vi "SPAN Stufen abfragen Gasteiler alle Komponenten.vi"(5 "GD LNI Cluster":T2, 6 "Sprachliste":string[][](array[string]), 7 "Boolsche Flags Cluster":T13, 8 "error in (no error)":errorcluster caption="Fehler (Eingang, kein Fehler)", 9 "Referenzen Cluster":T12, 10 "SPAN Index in":i32, 11 "SpanInletClusterArray in":T3[](array[typedef]) {"zusätzliche Zeitdauer Erster Punkt" min=30 step=1 format="%#_5g"; "Zeitdauer Stufen" format="%#_5g"; "Max Fehler" format="%#_5g"; "Anzahl Stufen" format="%#_5g"; "Komponenten"."Komponente 5"."Komponente:" items=["NO (350,3000) LP 191C", "NO2 (150) LP 191C (1of2)", "NO2 (2000) LP 191C (2of2)", "N2O (300) LP 191C (1of2)", "NH3 (300) LP 191C (1of2)", "NH3 (900,3000) LP 191C (2of2)", "HNCO (400) 191C", "H2O% (30) LP 191C", "Formaldehyde (70,500) LP 191C", "CO2 low% (4) LP 191C (2of2)", "CO2% (20) LP 191C (1of2)", "CO (700) LP 191C (1of3)", "CO% (1) LP 191C (2of3)", "Propylene (1000) LP 191C", "Aromatic HC C7 (500) LP 191C", "Ethylene (1000) LP 191C", "CH4 (250) LP 191C (1of2)", "CH4 (5000) LP 191C (2of2)", "Ethane (1000) LP 191C", "Acetylene (1000) LP 191C", "HNO2 (20) 191C", "MeOH (1000) 191C", "CO% (10) LP 191C (3of3)", "Formic Acid (100) 191C", "SO2 (500) LP 191C", "Acetaldehyde (1000) LP 191C", "COS (100) LP 191C", "1,3 butadiene (100) LP 191C", "Oil as Octane (200) LP 191C", "N2O (1000) LP 191C (2of2)", "Propane (200) LP 191C", "NO2 autorange (2000)", "CO autorange (100000)", "CH4 autorange (5000)", "NH3 autorange (3000)", "Temp. Gascell", "Pressure Gascell", "sBeam@2500"]; "Komponenten"."Komponente 5"."Konzentration IST" format="%#.4f"; "Komponenten"."Komponente 5"."Genauigkeit" format="%#.1f"; "Komponenten"."Komponente 4"."Komponente:" items=["NO (350,3000) LP 191C", "NO2 (150) LP 191C (1of2)", "NO2 (2000) LP 191C (2of2)", "N2O (300) LP 191C (1of2)", "NH3 (300) LP 191C (1of2)", "NH3 (900,3000) LP 191C (2of2)", "HNCO (400) 191C", "H2O% (30) LP 191C", "Formaldehyde (70,500) LP 191C", "CO2 low% (4) LP 191C (2of2)", "CO2% (20) LP 191C (1of2)", "CO (700) LP 191C (1of3)", "CO% (1) LP 191C (2of3)", "Propylene (1000) LP 191C", "Aromatic HC C7 (500) LP 191C", "Ethylene (1000) LP 191C", "CH4 (250) LP 191C (1of2)", "CH4 (5000) LP 191C (2of2)", "Ethane (1000) LP 191C", "Acetylene (1000) LP 191C", "HNO2 (20) 191C", "MeOH (1000) 191C", "CO% (10) LP 191C (3of3)", "Formic Acid (100) 191C", "SO2 (500) LP 191C", "Acetaldehyde (1000) LP 191C", "COS (100) LP 191C", "1,3 butadiene (100) LP 191C", "Oil as Octane (200) LP 191C", "N2O (1000) LP 191C (2of2)", "Propane (200) LP 191C", "NO2 autorange (2000)", "CO autorange (100000)", "CH4 autorange (5000)", "NH3 autorange (3000)", "Temp. Gascell", "Pressure Gascell", "sBeam@2500"]; "Komponenten"."Komponente 4"."Konzentration IST" format="%#.4f"; "Komponenten"."Komponente 4"."Genauigkeit" format="%#.1f"; "Komponenten"."Komponente 3"."Komponente:" items=["NO (350,3000) LP 191C", "NO2 (150) LP 191C (1of2)", "NO2 (2000) LP 191C (2of2)", "N2O (300) LP 191C (1of2)", "NH3 (300) LP 191C (1of2)", "NH3 (900,3000) LP 191C (2of2)", "HNCO (400) 191C", "H2O% (30) LP 191C", "Formaldehyde (70,500) LP 191C", "CO2 low% (4) LP 191C (2of2)", "CO2% (20) LP 191C (1of2)", "CO (700) LP 191C (1of3)", "CO% (1) LP 191C (2of3)", "Propylene (1000) LP 191C", "Aromatic HC C7 (500) LP 191C", "Ethylene (1000) LP 191C", "CH4 (250) LP 191C (1of2)", "CH4 (5000) LP 191C (2of2)", "Ethane (1000) LP 191C", "Acetylene (1000) LP 191C", "HNO2 (20) 191C", "MeOH (1000) 191C", "CO% (10) LP 191C (3of3)", "Formic Acid (100) 191C", "SO2 (500) LP 191C", "Acetaldehyde (1000) LP 191C", "COS (100) LP 191C", "1,3 butadiene (100) LP 191C", "Oil as Octane (200) LP 191C", "N2O (1000) LP 191C (2of2)", "Propane (200) LP 191C", "NO2 autorange (2000)", "CO autorange (100000)", "CH4 autorange (5000)", "NH3 autorange (3000)", "Temp. Gascell", "Pressure Gascell", "sBeam@2500"]; "Komponenten"."Komponente 3"."Konzentration IST" format="%#.4f"; "Komponenten"."Komponente 3"."Genauigkeit" format="%#.1f"; "Komponenten"."Komponente 2"."Komponente:" items=["NO (350,3000) LP 191C", "NO2 (150) LP 191C (1of2)", "NO2 (2000) LP 191C (2of2)", "N2O (300) LP 191C (1of2)", "NH3 (300) LP 191C (1of2)", "NH3 (900,3000) LP 191C (2of2)", "HNCO (400) 191C", "H2O% (30) LP 191C", "Formaldehyde (70,500) LP 191C", "CO2 low% (4) LP 191C (2of2)", "CO2% (20) LP 191C (1of2)", "CO (700) LP 191C (1of3)", "CO% (1) LP 191C (2of3)", "Propylene (1000) LP 191C", "Aromatic HC C7 (500) LP 191C", "Ethylene (1000) LP 191C", "CH4 (250) LP 191C (1of2)", "CH4 (5000) LP 191C (2of2)", "Ethane (1000) LP 191C", "Acetylene (1000) LP 191C", "HNO2 (20) 191C", "MeOH (1000) 191C", "CO% (10) LP 191C (3of3)", "Formic Acid (100) 191C", "SO2 (500) LP 191C", "Acetaldehyde (1000) LP 191C", "COS (100) LP 191C", "1,3 butadiene (100) LP 191C", "Oil as Octane (200) LP 191C", "N2O (1000) LP 191C (2of2)", "Propane (200) LP 191C", "NO2 autorange (2000)", "CO autorange (100000)", "CH4 autorange (5000)", "NH3 autorange (3000)", "Temp. Gascell", "Pressure Gascell", "sBeam@2500"]; "Komponenten"."Komponente 2"."Konzentration IST" format="%#.4f"; "Komponenten"."Komponente 2"."Genauigkeit" format="%#.1f"; "Komponenten"."Komponente 1"."Komponente:" items=["NO (350,3000) LP 191C", "NO2 (150) LP 191C (1of2)", "NO2 (2000) LP 191C (2of2)", "N2O (300) LP 191C (1of2)", "NH3 (300) LP 191C (1of2)", "NH3 (900,3000) LP 191C (2of2)", "HNCO (400) 191C", "H2O% (30) LP 191C", "Formaldehyde (70,500) LP 191C", "CO2 low% (4) LP 191C (2of2)", "CO2% (20) LP 191C (1of2)", "CO (700) LP 191C (1of3)", "CO% (1) LP 191C (2of3)", "Propylene (1000) LP 191C", "Aromatic HC C7 (500) LP 191C", "Ethylene (1000) LP 191C", "CH4 (250) LP 191C (1of2)", "CH4 (5000) LP 191C (2of2)", "Ethane (1000) LP 191C", "Acetylene (1000) LP 191C", "HNO2 (20) 191C", "MeOH (1000) 191C", "CO% (10) LP 191C (3of3)", "Formic Acid (100) 191C", "SO2 (500) LP 191C", "Acetaldehyde (1000) LP 191C", "COS (100) LP 191C", "1,3 butadiene (100) LP 191C", "Oil as Octane (200) LP 191C", "N2O (1000) LP 191C (2of2)", "Propane (200) LP 191C", "NO2 autorange (2000)", "CO autorange (100000)", "CH4 autorange (5000)", "NH3 autorange (3000)", "Temp. Gascell", "Pressure Gascell", "sBeam@2500"]; "Komponenten"."Komponente 1"."Konzentration IST" format="%#.4f"; "Komponenten"."Komponente 1"."Genauigkeit" format="%#.1f"; "Ablaufdatum" format="%<%d.%m.%Y>T"; "Gasflasche" items=["----"=10000, "IAG NH3 3000"=0, "IAG NH3 200"=1, "IAG NH3 2000"=2, "IAG MG"=3, "IAG O2"=4]}) -> (0 "error out":errorcluster, 1 "Component Index out":i32, 2 "SPAN Index out":i32, 3 "SpanInletClusterArray out":T3[](array[typedef]) {"zusätzliche Zeitdauer Erster Punkt" min=30 step=1 format="%#_5g"; "Zeitdauer Stufen" format="%#_5g"; "Max Fehler" format="%#_5g"; "Anzahl Stufen" format="%#_5g"; "Komponenten"."Komponente 5"."Komponente:" items=["NO (350,3000) LP 191C", "NO2 (150) LP 191C (1of2)", "NO2 (2000) LP 191C (2of2)", "N2O (300) LP 191C (1of2)", "NH3 (300) LP 191C (1of2)", "NH3 (900,3000) LP 191C (2of2)", "HNCO (400) 191C", "H2O% (30) LP 191C", "Formaldehyde (70,500) LP 191C", "CO2 low% (4) LP 191C (2of2)", "CO2% (20) LP 191C (1of2)", "CO (700) LP 191C (1of3)", "CO% (1) LP 191C (2of3)", "Propylene (1000) LP 191C", "Aromatic HC C7 (500) LP 191C", "Ethylene (1000) LP 191C", "CH4 (250) LP 191C (1of2)", "CH4 (5000) LP 191C (2of2)", "Ethane (1000) LP 191C", "Acetylene (1000) LP 191C", "HNO2 (20) 191C", "MeOH (1000) 191C", "CO% (10) LP 191C (3of3)", "Formic Acid (100) 191C", "SO2 (500) LP 191C", "Acetaldehyde (1000) LP 191C", "COS (100) LP 191C", "1,3 butadiene (100) LP 191C", "Oil as Octane (200) LP 191C", "N2O (1000) LP 191C (2of2)", "Propane (200) LP 191C", "NO2 autorange (2000)", "CO autorange (100000)", "CH4 autorange (5000)", "NH3 autorange (3000)", "Temp. Gascell", "Pressure Gascell", "sBeam@2500"]; "Komponenten"."Komponente 5"."Konzentration IST" format="%#.4f"; "Komponenten"."Komponente 5"."Genauigkeit" format="%#.1f"; "Komponenten"."Komponente 4"."Komponente:" items=["NO (350,3000) LP 191C", "NO2 (150) LP 191C (1of2)", "NO2 (2000) LP 191C (2of2)", "N2O (300) LP 191C (1of2)", "NH3 (300) LP 191C (1of2)", "NH3 (900,3000) LP 191C (2of2)", "HNCO (400) 191C", "H2O% (30) LP 191C", "Formaldehyde (70,500) LP 191C", "CO2 low% (4) LP 191C (2of2)", "CO2% (20) LP 191C (1of2)", "CO (700) LP 191C (1of3)", "CO% (1) LP 191C (2of3)", "Propylene (1000) LP 191C", "Aromatic HC C7 (500) LP 191C", "Ethylene (1000) LP 191C", "CH4 (250) LP 191C (1of2)", "CH4 (5000) LP 191C (2of2)", "Ethane (1000) LP 191C", "Acetylene (1000) LP 191C", "HNO2 (20) 191C", "MeOH (1000) 191C", "CO% (10) LP 191C (3of3)", "Formic Acid (100) 191C", "SO2 (500) LP 191C", "Acetaldehyde (1000) LP 191C", "COS (100) LP 191C", "1,3 butadiene (100) LP 191C", "Oil as Octane (200) LP 191C", "N2O (1000) LP 191C (2of2)", "Propane (200) LP 191C", "NO2 autorange (2000)", "CO autorange (100000)", "CH4 autorange (5000)", "NH3 autorange (3000)", "Temp. Gascell", "Pressure Gascell", "sBeam@2500"]; "Komponenten"."Komponente 4"."Konzentration IST" format="%#.4f"; "Komponenten"."Komponente 4"."Genauigkeit" format="%#.1f"; "Komponenten"."Komponente 3"."Komponente:" items=["NO (350,3000) LP 191C", "NO2 (150) LP 191C (1of2)", "NO2 (2000) LP 191C (2of2)", "N2O (300) LP 191C (1of2)", "NH3 (300) LP 191C (1of2)", "NH3 (900,3000) LP 191C (2of2)", "HNCO (400) 191C", "H2O% (30) LP 191C", "Formaldehyde (70,500) LP 191C", "CO2 low% (4) LP 191C (2of2)", "CO2% (20) LP 191C (1of2)", "CO (700) LP 191C (1of3)", "CO% (1) LP 191C (2of3)", "Propylene (1000) LP 191C", "Aromatic HC C7 (500) LP 191C", "Ethylene (1000) LP 191C", "CH4 (250) LP 191C (1of2)", "CH4 (5000) LP 191C (2of2)", "Ethane (1000) LP 191C", "Acetylene (1000) LP 191C", "HNO2 (20) 191C", "MeOH (1000) 191C", "CO% (10) LP 191C (3of3)", "Formic Acid (100) 191C", "SO2 (500) LP 191C", "Acetaldehyde (1000) LP 191C", "COS (100) LP 191C", "1,3 butadiene (100) LP 191C", "Oil as Octane (200) LP 191C", "N2O (1000) LP 191C (2of2)", "Propane (200) LP 191C", "NO2 autorange (2000)", "CO autorange (100000)", "CH4 autorange (5000)", "NH3 autorange (3000)", "Temp. Gascell", "Pressure Gascell", "sBeam@2500"]; "Komponenten"."Komponente 3"."Konzentration IST" format="%#.4f"; "Komponenten"."Komponente 3"."Genauigkeit" format="%#.1f"; "Komponenten"."Komponente 2"."Komponente:" items=["NO (350,3000) LP 191C", "NO2 (150) LP 191C (1of2)", "NO2 (2000) LP 191C (2of2)", "N2O (300) LP 191C (1of2)", "NH3 (300) LP 191C (1of2)", "NH3 (900,3000) LP 191C (2of2)", "HNCO (400) 191C", "H2O% (30) LP 191C", "Formaldehyde (70,500) LP 191C", "CO2 low% (4) LP 191C (2of2)", "CO2% (20) LP 191C (1of2)", "CO (700) LP 191C (1of3)", "CO% (1) LP 191C (2of3)", "Propylene (1000) LP 191C", "Aromatic HC C7 (500) LP 191C", "Ethylene (1000) LP 191C", "CH4 (250) LP 191C (1of2)", "CH4 (5000) LP 191C (2of2)", "Ethane (1000) LP 191C", "Acetylene (1000) LP 191C", "HNO2 (20) 191C", "MeOH (1000) 191C", "CO% (10) LP 191C (3of3)", "Formic Acid (100) 191C", "SO2 (500) LP 191C", "Acetaldehyde (1000) LP 191C", "COS (100) LP 191C", "1,3 butadiene (100) LP 191C", "Oil as Octane (200) LP 191C", "N2O (1000) LP 191C (2of2)", "Propane (200) LP 191C", "NO2 autorange (2000)", "CO autorange (100000)", "CH4 autorange (5000)", "NH3 autorange (3000)", "Temp. Gascell", "Pressure Gascell", "sBeam@2500"]; "Komponenten"."Komponente 2"."Konzentration IST" format="%#.4f"; "Komponenten"."Komponente 2"."Genauigkeit" format="%#.1f"; "Komponenten"."Komponente 1"."Komponente:" items=["NO (350,3000) LP 191C", "NO2 (150) LP 191C (1of2)", "NO2 (2000) LP 191C (2of2)", "N2O (300) LP 191C (1of2)", "NH3 (300) LP 191C (1of2)", "NH3 (900,3000) LP 191C (2of2)", "HNCO (400) 191C", "H2O% (30) LP 191C", "Formaldehyde (70,500) LP 191C", "CO2 low% (4) LP 191C (2of2)", "CO2% (20) LP 191C (1of2)", "CO (700) LP 191C (1of3)", "CO% (1) LP 191C (2of3)", "Propylene (1000) LP 191C", "Aromatic HC C7 (500) LP 191C", "Ethylene (1000) LP 191C", "CH4 (250) LP 191C (1of2)", "CH4 (5000) LP 191C (2of2)", "Ethane (1000) LP 191C", "Acetylene (1000) LP 191C", "HNO2 (20) 191C", "MeOH (1000) 191C", "CO% (10) LP 191C (3of3)", "Formic Acid (100) 191C", "SO2 (500) LP 191C", "Acetaldehyde (1000) LP 191C", "COS (100) LP 191C", "1,3 butadiene (100) LP 191C", "Oil as Octane (200) LP 191C", "N2O (1000) LP 191C (2of2)", "Propane (200) LP 191C", "NO2 autorange (2000)", "CO autorange (100000)", "CH4 autorange (5000)", "NH3 autorange (3000)", "Temp. Gascell", "Pressure Gascell", "sBeam@2500"]; "Komponenten"."Komponente 1"."Konzentration IST" format="%#.4f"; "Komponenten"."Komponente 1"."Genauigkeit" format="%#.1f"; "Ablaufdatum" format="%<%d.%m.%Y>T"; "Gasflasche" items=["----"=10000, "IAG NH3 3000"=0, "IAG NH3 200"=1, "IAG NH3 2000"=2, "IAG MG"=3, "IAG O2"=4]}, 4 "Anzahl Stufen":sgl)   [LabVIEW 2020, in "Linearisierung v2.lvlib" / "SpanEinstellungen.lvlib"]
uses:
  SpanEinstellungen.lvlib
  SpanInletCluster.ctl
  Seiten/System Einstellungen V2/Konfig Gasflasche.ctl
  Seiten/System Einstellungen V2/Analysatoren.ctl
  Seiten/System Einstellungen V2/Gasflasche Auswahl.ctl
  Komponentencluster mit Formel.ctl
  Komponentenauswahl mit Formel.ctl
  Visualisierungs Elemente/String - Eingabefeld.ctl
  Einheit.ctl
  Seiten/System Einstellungen V2/Traegergas.ctl
  Boolsche Stufen Flags.ctl
  GD Abfrage Referenzen.ctl
  Visualisierungs Elemente/Checkbox(boolsch).ctl
  Aktion FGV SPAN Verriegelung.ctl
  Linearisierung v2.lvlib
  Gasteiler/Gasteiler.lvlib
  Seiten/System Einstellungen V2/System Einstellungen V2.lvlib
panel:
  # "sec"
  # "%"
  # "sec"
  # "Komponente"
  # "Formel"
  # "Konzentration"
  # "Einheit"
  # "Genauigkeit [%]"
  # "sec"
  # "%"
  # "sec"
  # "Komponente"
  # "Formel"
  # "Konzentration"
  # "Einheit"
  # "Genauigkeit [%]"
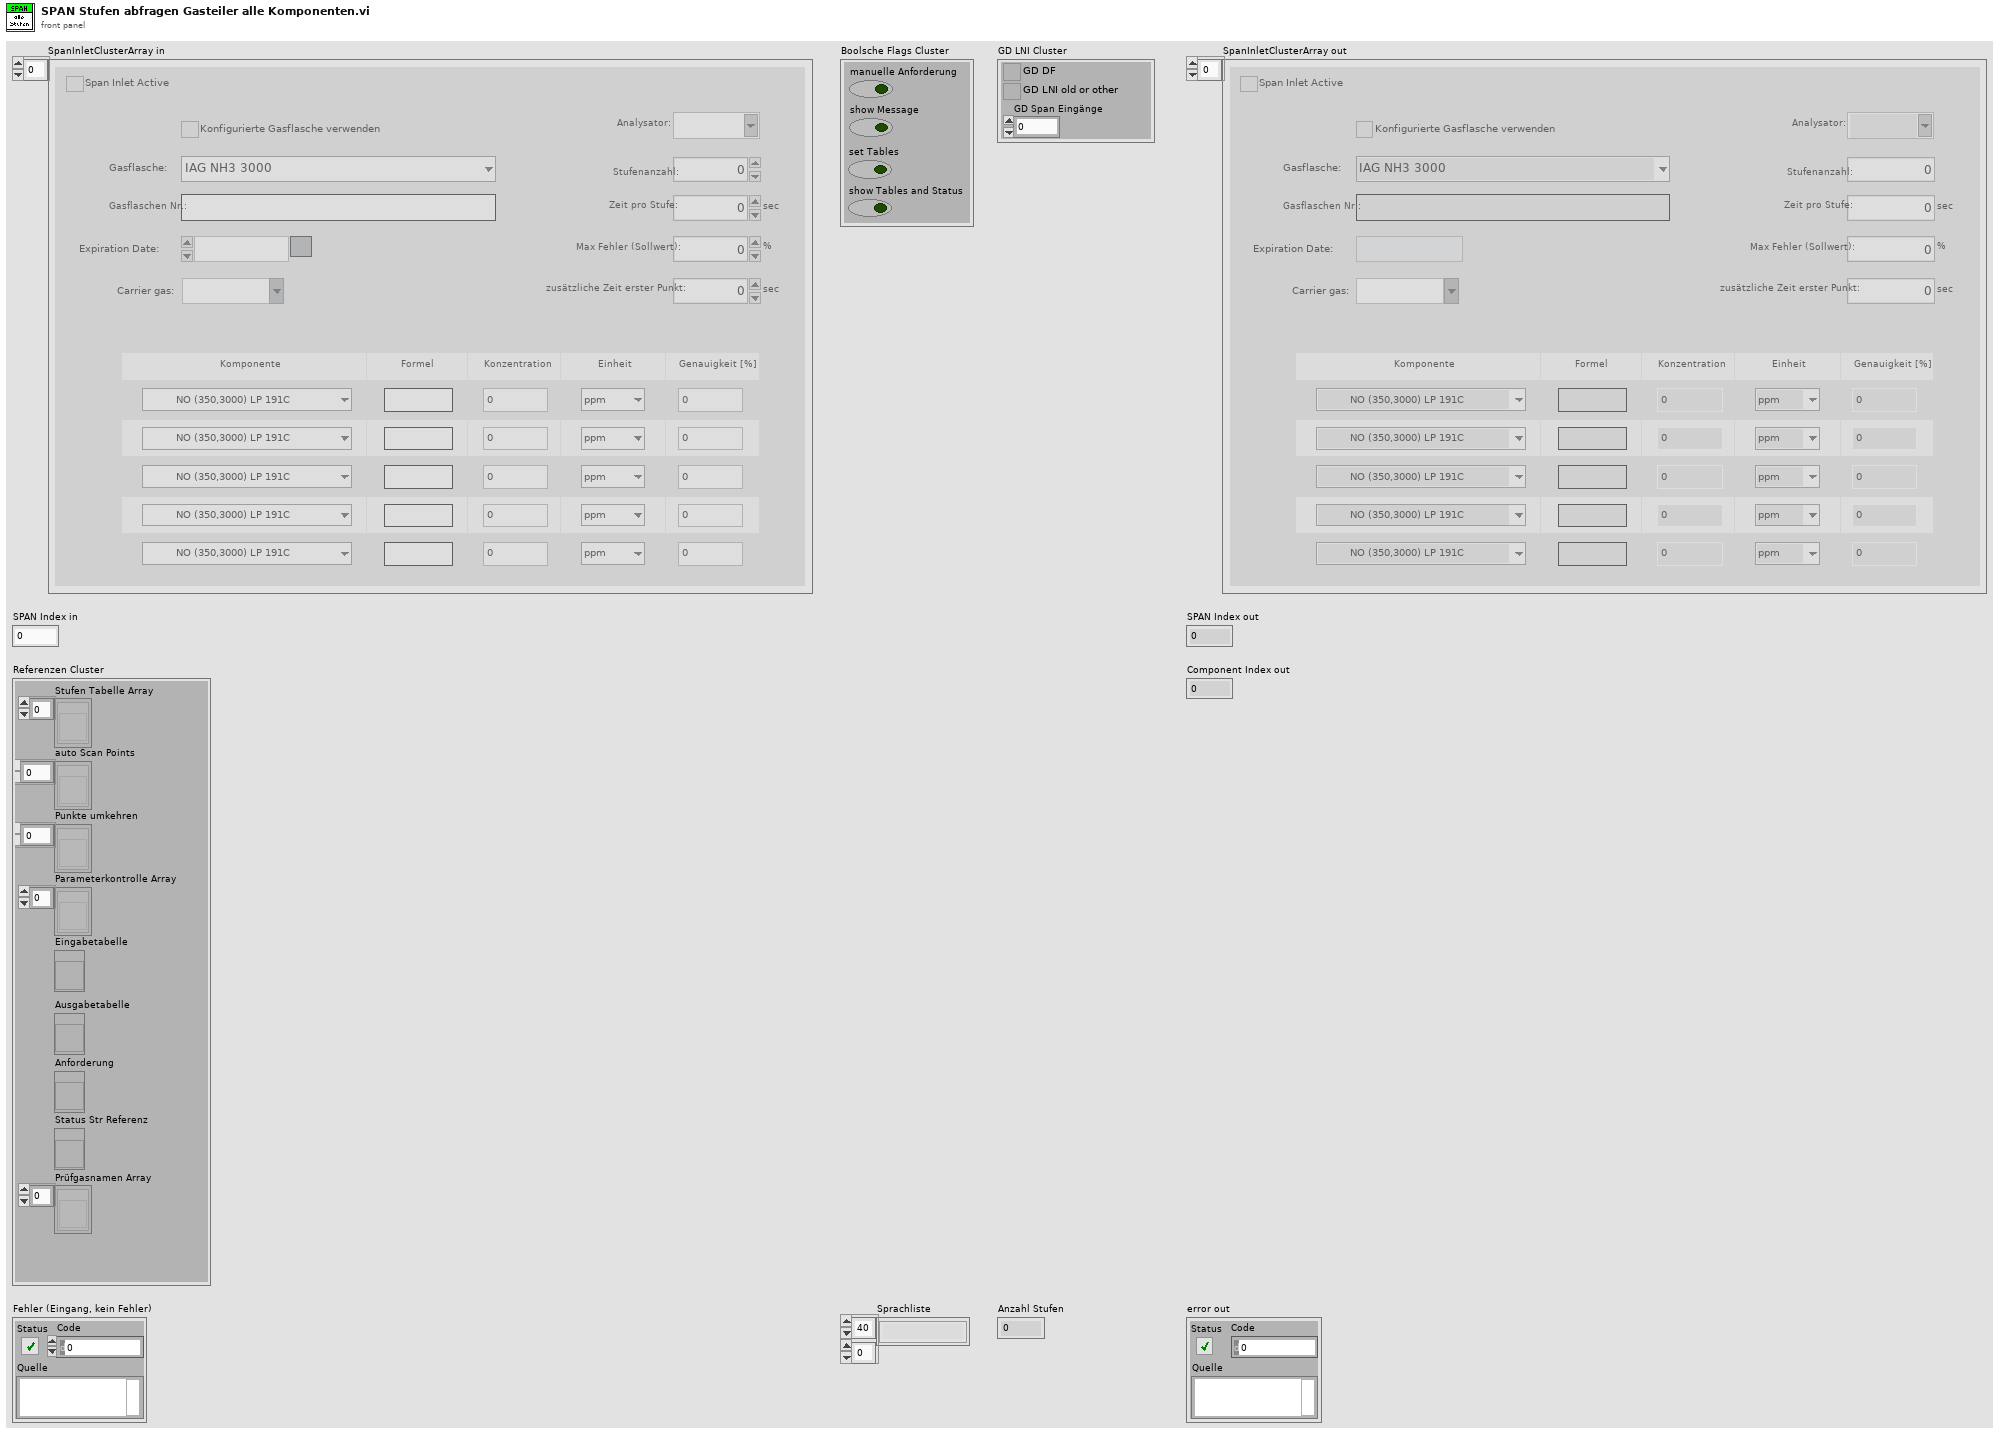
[diagram p1: front panel]
types:
  T1 = typedef "Checkbox(boolsch).ctl" = bool
  T2 = cluster{"GD DF":T1, "GD LNI old or other":T1, "GD Span Eingänge":u16}
  T3 = typedef "Linearisierung v2.lvlib/SpanEinstellungen.lvlib/SpanInletCluster.ctl" = cluster{"Span Inlet Active":T4, "Analysator":T5, "Konfig Gasflasche":T4, "Gasflasche":T6, "Gasflaschen Nr.:":string, "Ablaufdatum":timestamp, "Komponenten":T7, "Zeitdauer Stufen":sgl, "Max Fehler":sgl, "Anzahl Stufen":sgl, "Trägergas":T11, "zusätzliche Zeitdauer Erster Punkt":sgl}
  T4 = typedef "System Einstellungen V2.lvlib/Konfig Gasflasche.ctl" = bool
  T5 = typedef "System Einstellungen V2.lvlib/Analysatoren.ctl" = string
  T6 = typedef "System Einstellungen V2.lvlib/Gasflasche Auswahl.ctl" = u16
  T7 = typedef "Linearisierung v2.lvlib/SpanEinstellungen.lvlib/Komponentencluster mit Formel.ctl" = cluster{"Komponente 1":T8, "Komponente 2":T8, "Komponente 3":T8, "Komponente 4":T8, "Komponente 5":T8}
  T8 = typedef "Linearisierung v2.lvlib/SpanEinstellungen.lvlib/Komponentenauswahl mit Formel.ctl" = cluster{"Komponente:":u16, "Summenformel":T9, "Konzentration IST":dbl, "Einheit":T10, "Genauigkeit":dbl}
  T9 = typedef "String - Eingabefeld.ctl" = string
  T10 = typedef "Linearisierung v2.lvlib/SpanEinstellungen.lvlib/Einheit.ctl" = enum16{"ppm", "%"}
  T11 = typedef "System Einstellungen V2.lvlib/Traegergas.ctl" = string
  T12 = typedef "Linearisierung v2.lvlib/SpanEinstellungen.lvlib/GD Abfrage Referenzen.ctl" = cluster{"Stufen Tabelle Array":refnum<vi>[], "auto Scan Points":refnum<vi>[], "Punkte umkehren":refnum<vi>[], "Parameterkontrolle Array":refnum<vi>[], "Eingabetabelle":refnum<vi>, "Ausgabetabelle":refnum<vi>, "Anforderung":refnum<vi>, "Status Str Referenz":refnum<vi>, "Prüfgasnamen Array":refnum<vi>[]}
  T13 = typedef "Linearisierung v2.lvlib/SpanEinstellungen.lvlib/Boolsche Stufen Flags.ctl" = cluster{"manuelle Anforderung":bool, "show Message":bool, "set Tables":bool, "show Tables and Status":bool}
  T14 = cluster{"GD LNI old or other":T1, "Index out":i32, "Component Index out":i32[], "aktive Komponenten Indices additional":u16[], "GD Span Eingänge":u16, "Gesamtkonzentration":dbl, "höchste Konzentration Teilkomponente":dbl}
  T15 = cluster{"Stufen Tabelle Array":string[][][], "EKAG Array":string[]}
  T16 = typedef "Linearisierung v2.lvlib/SpanEinstellungen.lvlib/Aktion FGV SPAN Verriegelung.ctl" = enum16{"lesen", "setrefs", "setcomp", "lock", "unlock", "Set Save EPA redirect", "Reset Save EPA redirect", "Set Postprocessing PDF", "Reset Postprocessing PDF", "Set Start Postprocessing PDF", "Reset Start Postprocessing PDF"}
  T17 = typedef "Linearisierung v2.lvlib/Auswahl Polynom Ordnung.ctl" = enum16{"autom.", "raw", "actual", "1", "2", "3", "4"}
  T18 = typedef "Linearisierung v2.lvlib/EPA Optionsfeld.ctl" = enum32{"Istwert", "Rohwert", "Linearisierter Wert"}
  T19 = cluster{"Component":cluster{"Component Name":string, "Component":u8, "Component Unit":string}, "Daten aufzeichnen Offset Cluster":cluster{"Autorange Offsets":string, "Autorange Spanfactors":string, "Polynome":cluster{"Polynome[0]":dbl, "Polynome[1]":dbl, "Polynome[2]":dbl, "Polynome[3]":dbl, "Polynome[4]":dbl}}, "Lin Offset Cluster":cluster{"Autorange Offsets":string, "Autorange Spanfactors":string, "Polynome":cluster{"Polynome[0]":dbl, "Polynome[1]":dbl, "Polynome[2]":dbl, "Polynome[3]":dbl, "Polynome[4]":dbl}, "Polynom-Ordnung":T17}, "EPA Optionsfeld":T18}
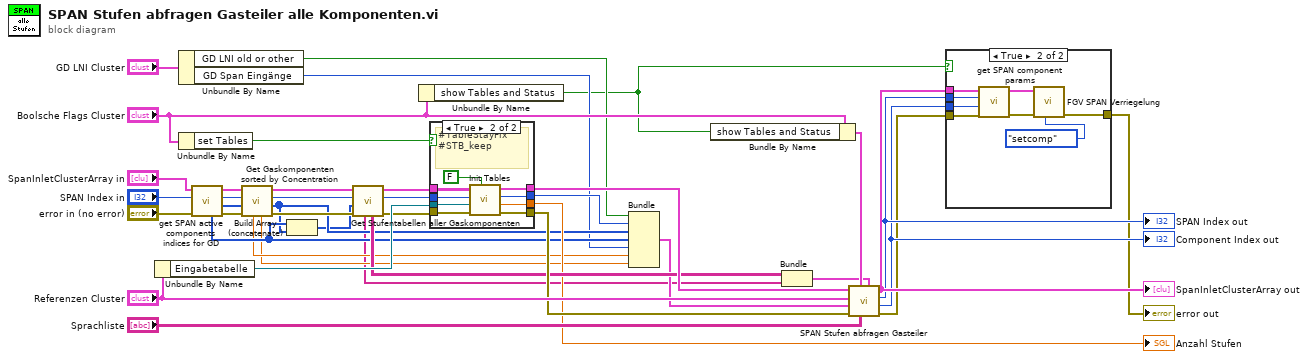
[diagram p0: block diagram]
diagram:
  n1 = Unbundle By Name("Referenzen Cluster") -> ("Eingabetabelle"=w35:refnum<vi>)
  n2 = Unbundle By Name("GD LNI Cluster") -> ("GD LNI old or other"=w12:T1, "GD Span Eingänge"=w11:u16)
  n3 = Unbundle By Name("Boolsche Flags Cluster") -> ("set Tables"=w33:bool)
  n4 = call "get SPAN active components indices for GD.vi"("error in (no error)"="error in (no error)", "SPAN Idx"="SPAN Index in", "SpanInletClusterArray in"="SpanInletClusterArray in") -> ("error out"=w20:errorcluster, "aktive Komponenten GD Indices"=w21:i32[], "SPAN Idx out"=w23:i32, "SpanInletClusterArray out"=w25:T3[], "aktive Komponenten Indices additional"=w16:u16[])  [unwired: 1 in, 3 out]
  n5 = call "Get Gaskomponenten sorted by Concentration.vi"("Fehler (Eingang, kein Fehler)"=w20, "Component Index"=w21, "SPAN Idx in (Eingang)"=w23, "SpanInletClusterArray in (Eingang)"=w25) -> ("Fehler (Ausgang)"=w19:errorcluster, "Component Index out"=w15:i32[], "SPAN Idx out (Ausgang)"=w22:i32, "SpanInletClusterArray out (Ausgang)"=w24:T3[], "höchste Konzentration Teilkomponente"=w9:dbl, "Gesamtkonzentration"=w10:dbl)  [unwired: 2 in]
  n6 = Build Array (concatenate)(w16, w15) -> (w14:i32[])
  n7 = call "Get Stufentabellen aller Gaskomponenten.vi"("Fehler (Eingang, kein Fehler)"=w19, "Component Index"=w14, "SPAN Idx in (Eingang)"=w22, "SpanInletClusterArray in (Eingang)"=w24) -> ("Fehler (Ausgang)"=w28:errorcluster, "SPAN Idx out (Ausgang)"=w29:i32, "SpanInletClusterArray out (Ausgang)"=w31:T3[], "Stufen Tabelle Array"=w27:string[][][], "EKAG Array"=w1:string[])  [unwired: 2 in, 1 out]
  n8 = Unbundle By Name("Boolsche Flags Cluster") -> ("show Tables and Status"=w5:bool)
  n9 = case shown="True" w33 {
    tunnel: w31 -> [w44 w53]
    tunnel: [w44 w52] -> w30
    tunnel: w29 -> [w43 w51]
    tunnel: [w42 w50] -> w36
    tunnel: w35 -> [_ w49]
    tunnel: [w43 w48] -> w34
    tunnel: w28 -> [w42 w47]
    tunnel: [_ w46] -> w26
    frame False {
    }
    frame True {
      # "#TableStayFix\n#STB_keep"
      n10 = call "Init Tables.vi"("init ohne Stufen"=FALSE, "error in (no error)"=w47, "Eingabetabelle"=w49, "Index in"=w51, "SpanInletClusterArray in"=w53) -> ("error out"=w50:errorcluster, "Anzahl Stufen"=w46:sgl, "Index out"=w48:i32, "SpanInletCluster out"=w52:T3[])  [unwired: 3 in]
    }
  }
  "Anzahl Stufen" <- w26
  n11 = Bundle("GD LNI old or other"=w12, "Index out"=w34, "Component Index out"=w15, "aktive Komponenten Indices additional"=w16, "GD Span Eingänge"=w11, "Gesamtkonzentration"=w10, "höchste Konzentration Teilkomponente"=w9) -> (w18:T14)  [unwired: 1 in]
  n12 = Bundle By Name(cluster="Boolsche Flags Cluster", "show Tables and Status"=w5) -> (w17:T13)
  n13 = Bundle("Stufen Tabelle Array"=w27, "EKAG Array"=w1) -> (w2:T15)  [unwired: 1 in]
  n14 = call "SPAN Stufen abfragen Gasteiler.vi"("GD Info Cluster"=w2, "Sprachliste"="Sprachliste", "Boolsche Stufen Flags Cluster"=w17, "error in (no error)"=w36, "Index"=w18, "Referenzen Cluster"="Referenzen Cluster", "SpanInletClusterArray in"=w30) -> ("error out"=w4:errorcluster, "Component Index out"=w6:i32, "SPAN Index out"=w7:i32, "SpanInletClusterArray out"=w8:T3[])  [unwired: 1 out]
  "SpanInletClusterArray out" <- w8
  "SPAN Index out" <- w7
  "Component Index out" <- w6
  n15 = case shown="True" w5 {
    tunnel: w8 -> [_ w60]
    tunnel: w7 -> [_ w59]
    tunnel: w6 -> [_ w58]
    tunnel: w4 -> [w54 w56]
    tunnel: [w54 w61] -> w3
    frame False {
    }
    frame True {
      n16 = call "get SPAN component params.vi"("Fehler (Eingang)"=w56, "Comp Idx"=w58, "active SPAN Idx"=w59, "SpanInletClusterArray"=w60) -> ("Fehler (Ausgang)"=w55:errorcluster, "Component Cluster"=w57:T19)  [unwired: 6 in]
      n17 = call "FGV SPAN Verriegelung.vi"("aktion"=Aktion_FGV_SPAN_Verriegelung."setcomp", "Component Cluster"=w57, "error in (no error)"=w55) -> ("error out"=w61:errorcluster)  [unwired: 6 in, 2 out]
    }
  }
  "error out" <- w3
